vi "InitOdometry.vi"(1 "child_frame_id":string, 2 "frame_id":string) -> (0 "OmniDynamics out":T1)   [LabVIEW 2014]
uses:
  Odometry.ctl
  TwistCovariance.ctl
  <vilib>/Analysis/7linalg.llb/Create Special Real Matrix.vi
  <vilib>/Analysis/NI_AALPro.lvlib
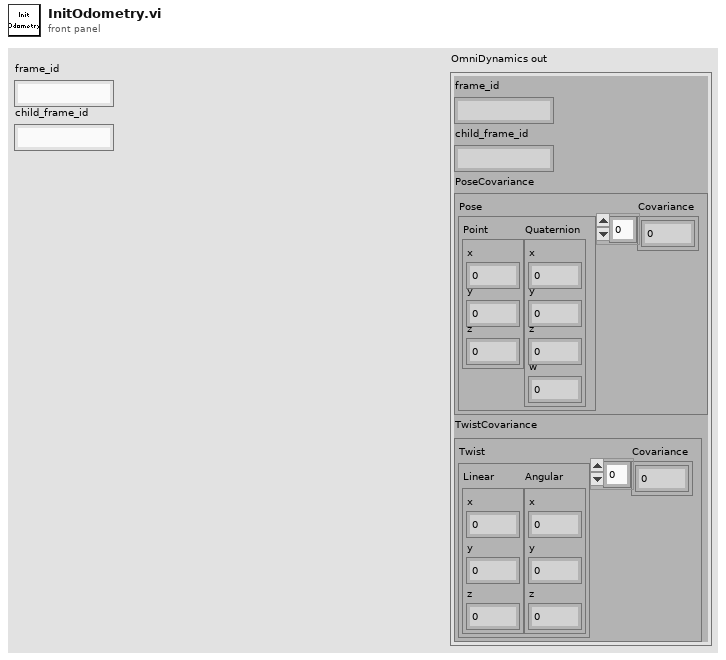
[diagram p1: front panel]
types:
  T1 = typedef "Odometry.ctl" = cluster{"frame_id":string, "child_frame_id":string, "PoseCovariance":cluster{"Pose":cluster{"Point":cluster{"x":dbl, "y":dbl, "z":dbl}, "Quaternion":cluster{"x":dbl, "y":dbl, "z":dbl, "w":dbl}}, "Covariance":dbl[]}, "TwistCovariance":T2}
  T2 = typedef "TwistCovariance.ctl" = cluster{"Twist":cluster{"Linear":cluster{"x":dbl, "y":dbl, "z":dbl}, "Angular":cluster{"x":dbl, "y":dbl, "z":dbl}}, "Covariance":dbl[]}
  T3 = cluster{"Linear":cluster{"x":dbl, "y":dbl, "z":dbl}, "Angular":cluster{"x":dbl, "y":dbl, "z":dbl}}
  T4 = cluster{"Point":cluster{"x":dbl, "y":dbl, "z":dbl}, "Quaternion":cluster{"x":dbl, "y":dbl, "z":dbl, "w":dbl}}
  T5 = typedef "NI_Matrix.lvlib/RealMatrix.ctl" = dbl[][]
  T6 = cluster{"Pose":cluster{"Point":cluster{"x":dbl, "y":dbl, "z":dbl}, "Quaternion":cluster{"x":dbl, "y":dbl, "z":dbl, "w":dbl}}, "Special Matrix":dbl[]}
  T7 = cluster{"Twist":cluster{"Linear":cluster{"x":dbl, "y":dbl, "z":dbl}, "Angular":cluster{"x":dbl, "y":dbl, "z":dbl}}, "Special Matrix":dbl[]}
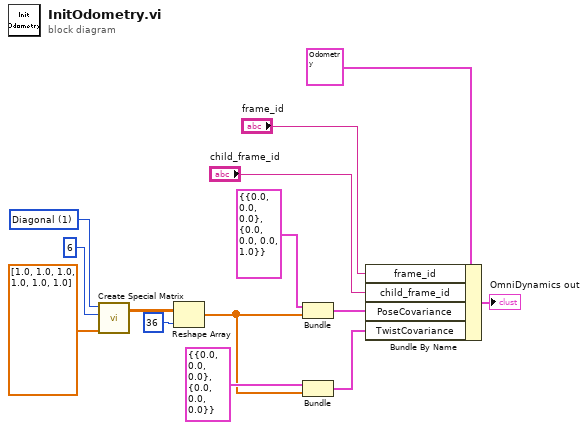
[diagram p0: block diagram]
diagram:
  w10 = 1 items=["Identity", "Diagonal", "Toeplitz", "Vandermonde", "Companion", "Hankel", "Hadamard", "Wilkinson", "Hilbert", "Inverse Hilbert", "Rosser", "Pascal"] ("matrix type")
  n1 = call-poly <vilib>:"Create Special Matrix.vi"("matrix type"=w10, "matrix size"=6, "Input Vector1"=dbl[] [1.0, 1.0, 1.0, 1.0, 1.0, 1.0]) -> ("Special Matrix"=w8:T5)  [unwired: 2 in, 1 out]
  n2 = Reshape Array(w8, 36 ("dimension size")) -> (w4:dbl[])
  n3 = Bundle("Pose"=T4 {"Point"={"x"=0.0, "y"=0.0, "z"=0.0}, "Quaternion"={"x"=0.0, "y"=0.0, "z"=0.0, "w"=1.0}}, "Special Matrix"=w4) -> (w6:T6)  [unwired: 1 in]
  n4 = Bundle("Twist"=T3 {"Linear"={"x"=0.0, "y"=0.0, "z"=0.0}, "Angular"={"x"=0.0, "y"=0.0, "z"=0.0}}, "Special Matrix"=w4) -> (w3:T7)  [unwired: 1 in]
  n5 = Bundle By Name(cluster=T1 {"frame_id"="", "child_frame_id"="", "PoseCovariance"={"Pose"={"Point"={"x"=0.0, "y"=0.0, "z"=0.0}, "Quaternion"={"x"=0.0, "y"=0.0, "z"=0.0, "w"=0.0}}, "Covariance"=[0.0, 0.0, 0.0, 0.0, 0.0]}, "TwistCovariance"={"Twist"={"Linear"={"x"=0.0, "y"=0.0, "z"=0.0}, "Angular"={"x"=0.0, "y"=0.0, "z"=0.0}}, "Covariance"=[0.0, 0.0, 0.0, 0.0, 0.0]}} ("OmniDynamics out"), "frame_id"="frame_id", "child_frame_id"="child_frame_id", "PoseCovariance"=w6, "TwistCovariance"=w3) -> (→"OmniDynamics out":T1)
